vi "AlliGator Get Decay Fit Parameter Map Data.vi"(0 "Multiple Decays Fit Parameters":dbl[][](array[numeric]), 1 "Compute Decay Fit Parameter Map":bool, 2 "Output ROI centers?":bool, 5 "X Resolution":i32, 7 "Y Resolution":i32, 11 "Error In":errorcluster, 12 "Map index":i32, 13 "Selected ROI Array":bool[](array[boolean])) -> (4 "Map Data (V x H)":dbl[][](array[numeric]), 6 "New Map Selected?":bool, 8 "# Filtered ROIs":i32, 10 "ROI Centers":cluster{"X":dbl, "Y":dbl}[](array[cluster]), 15 "Error Out":errorcluster)   [LabVIEW 2021, in "AlliGator Decay Fit Parameter Map.lvlib"]
doc: "Fills in matrix with fit parameter wherever it has been computed, NaN otherwise."
uses:
  AlliGator Decay Fit Parameter Map.lvlib
  Globals, Variables, Constants/AlliGator Variables List.ctl
  Variant/Variant to Data/Variant to Boolean.vi
  <vilib>/Utility/error.llb/Error Cluster From Error Code.vi
  <vilib>/ErrorRing/Error Ring.xnode
  Globals, Variables, Constants/AlliGator Globals, Variables & Constants.lvlib
  Variant/Variant to Data/Variant to Data.lvlib
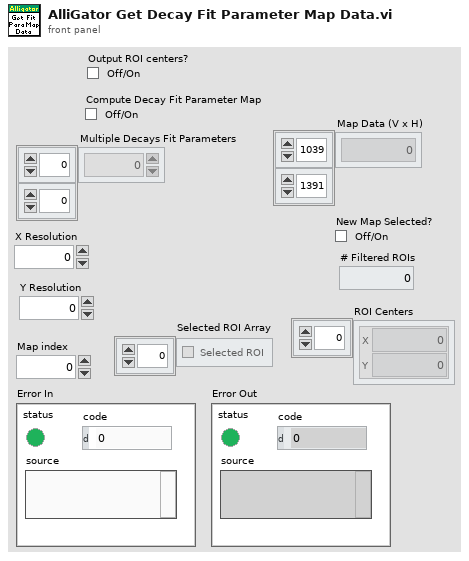
[diagram p1: front panel]
types:
  T1 = typedef "AlliGator Globals, Variables & Constants.lvlib/AlliGator Variables List.ctl" = enum16{"---- GUI ----", "GUI:Initialization Status", "GUI:State Indicators Refnum", "GUI:Original AlliGator Menu Items", "GUI:Current Action Loop State", "GUI:Script in progress", "GUI:Playback", "GUI:Loop Playback", "GUI:Search ROI Used", "GUI:Search ROI", "Decay Graph Max Legend Size", "Intensity Graph Max Legend Size", "Decay Statistics Graph Max Legend Size", "Phasor Graph Max Legend Size", "Phasor Ratio Graph Max Legend Size", "Lifetime Graph Max Legend Size", "---- Files ----", "Files:Export Dataset Frames as Individual Files", "Files:Show Batch Export Help Balloons", "Files:Frames in Dataset", "Files:ptu File Frame Start Indices", "Files:Current Frame in Dataset", "Files:Current Frame Timestamp", "Files:Dataset Loaded", "Files:Dataset Metadata", "Files:Dataset Channel", "Files:Dataset Data Description", "Files:Background Dataset Metadata", "Files:Background Dataset Channel", "Files:Background Dataset Data Description", "Files:Background File Subtraction", "Files:Background File Path", "Files:Background File Pile-up Correction", "Files:Background File Pixel Well Capacity", "Files:Background File Scaling Factor", "Files:Current Dataset Load Settings", "Files:Dataset Path", "Files:ICCD-specific Information", "Files:Macrotime Gate Separation", "------ Python Plugins ------", "Python Plugins:Information", "Python Plugins:Python Session", "Python Plugins:Valid Python Session?", "---- Source Image ----", "Source Image:ROIs", "Source Image:Current ROI", "Source Image:ROI Event Refnum", "X_Source Image:Display Range", "X_Source Image:Palette Information", "X_Source Image:Type of Displayed Image", "X_Time Gate Slider", "Source Image:Palette List", "Source Image:Scale", "Source Image:ROI Overlay Color", "Source Image:Overlay to Erase", "Source Image:Is Displayed Image Accumulated", "Source Image:White Light Image Modified", "Source Image:Mask Image Modified", "---- Image Profile Window ----", "Image Profile:Window Event Refnum", "Image Profile:IntensityType", "Image Profile:Intensity Average Type", "Image Profile:Intensity-weighted SDV", "Image Profile:Box Profile Type", "Image Profile:Window Open", "Image Profile:Plotted Fit Parameter", "------ Phasor Graph -------", "Phasor Graph:Show Line", "---- Phasor Plot ---", "Phasor Plot:Parameters Changed", "Phasor Plot:FLI Dataset Modified since last Calculation", "Phasor Harmonics Data", "Selected Phasor Harmonics", "Phasor Harmonic Manager Event Refnum", "Phasor Plot:ROIs", "Phasor Plot:Current ROI", "Phasor Plot:ROI Event Refnum", "Phasor Plot:Image Reference Points", "Phasor Plot:Computed", "Phasor Plot:Palette Information", "Phasor Plot:Palette List", "Phasor Plot:Phasor Ratio Palette Information", "Phasor Plot:Phasor Ratio Palette List", "Phasor Plot:Image Scale", "Phasor Plot:Image Overlay to Erase", "Phasor Plot:Image Elements to Update", "Phasor Plot:Current Calculation Parameters", "Phasor Plot:Current Calibration Options", "Phasor Plot:Reset Cumulated Phasor Plot", "Phasor Plot:Reference 1", "Phasor Plot:Lifetime Reference 1", "Phasor Plot:Reference 1 Frequency", "Phasor Plot:Reference 2", "Phasor Plot:Lifetime Reference 2", "Phasor Plot:Reference 2 Frequency", "---- Decay Analysis ----", "Number of Selected Decays to Fit", "LS Fit Results", "LAR Fit Results", "BS Fit Results", "Last Decay Max - Min", "Best Fit Parameters", "Best Fit Parameter Names", "Actual Size X", "Actual Size Y", "Binning X", "Binning Y", "Actual # Gates", "Dataset Number", "Gates to...", "Gates Skipped", "Gates to keep", "Gate Step", "Gate Separation", "Reversed Gates", "Pile-up Correction", "Pixel Well Capacity", "Background Subtracted", "Background Subtraction Method", "Background Definition Range", "Background File (deprecated)", "Number of Dataset Accumulated", "Array of Accumulated Dataset Paths", "Do Averaged Datasets", "Destination File Path", "Process Plot Target", "Use 1/D as Phasor Frequency", "---- Decay Fit Parameter Map -----", "Decay Fit Parameter Map:Palette Information", "Decay Fit Parameter Map:Palette List", "Decay Fit Parameter Map:X Resolution", "Decay Fit Parameter Map:Y Resolution", "Decay Fit Parameter Map:Use Decay Fit Result Constraints", "Decay Fit Parameter Map:Decay Fit Result Constraints", "Decay Fit Parameter Map:Decay Fit Result Constraints Applied", "---- Parameter Map ----", "Parameter Map:Palette Information", "Parameter Map:Palette List", "------- Local Decay Window ---------", "Local Decay Graph Window:Event Refnum", "Local Decay Graph Window:Use normalized IRF for convolution", "----- Miscellaneous ----", "Misc:Skippable Dialog Windows Status"}
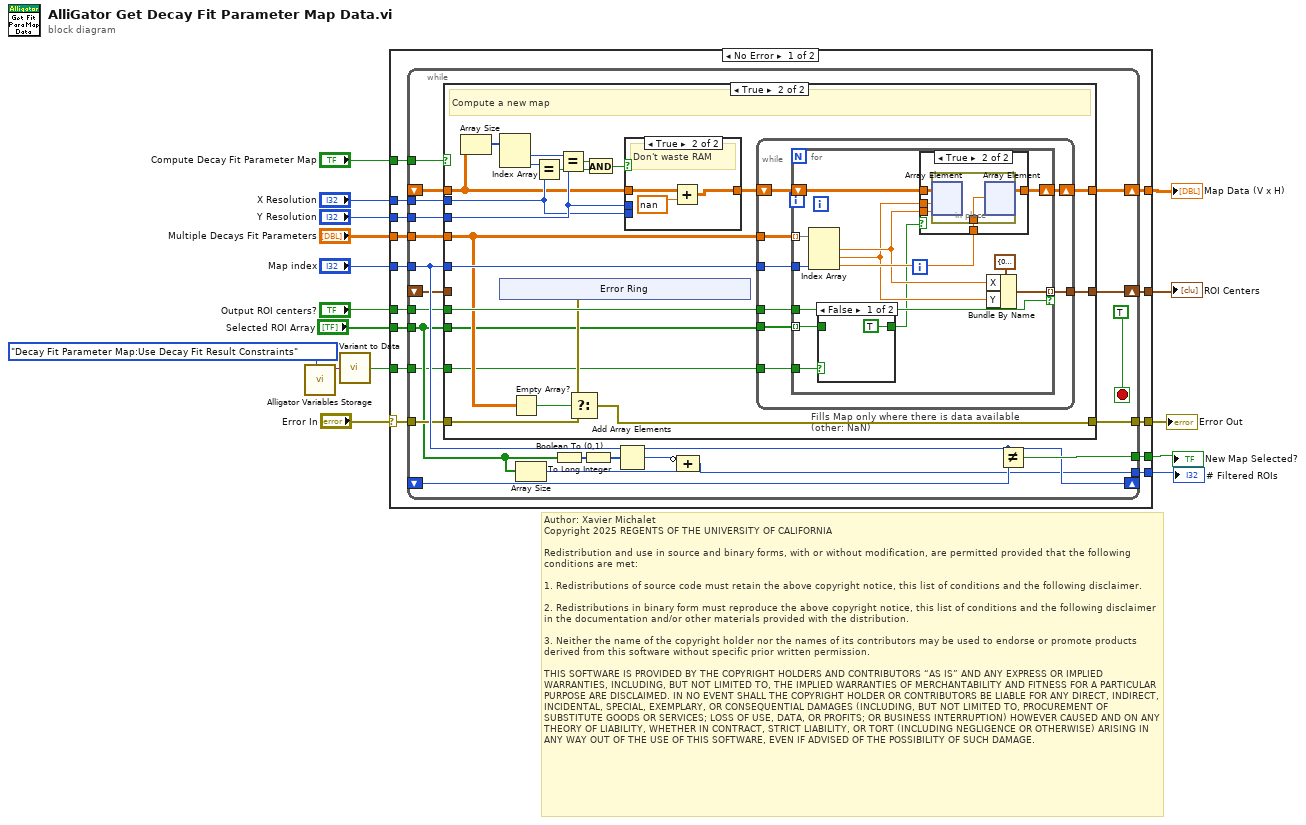
[diagram p0: block diagram]
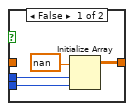
[diagram p5: hidden frame]
diagram:
  # "Author: Xavier Michalet\nCopyright 2025 REGENTS OF THE UNIVERSITY OF CALIFORNIA\n\nRedistribution and use in source and binary forms, with or without modification, are permitted provided that the following conditions are met:\n\n1. Redistributions of source code must retain the above copyright notice, this list of conditions and the following disclaimer.\n\n2. Redistributions in binary form must reproduce the above copyright notice, this list of conditions and the following disclaimer in the documentation and/or other materials provided with the distribution.\n\n3. Neither the name of the copyright holder nor the names of its contributors may be used to endorse or promote products derived from this software without specific prior written permission.\n\nTHIS SOFTWARE IS PROVIDED BY THE COPYRIGHT HOLDERS AND CONTRIBUTORS “AS IS” AND ANY EXPRESS OR IMPLIED WARRANTIES, INCLUDING, BUT NOT LIMITED TO, THE IMPLIED WARRANTIES OF MERCHANTABILITY AND FITNESS FOR A PARTICULAR PURPOSE ARE DISCLAIMED. IN NO EVENT SHALL THE COPYRIGHT HOLDER OR CONTRIBUTORS BE LIABLE FOR ANY DIRECT, INDIRECT, INCIDENTAL, SPECIAL, EXEMPLARY, OR CONSEQUENTIAL DAMAGES (INCLUDING, BUT NOT LIMITED TO, PROCUREMENT OF SUBSTITUTE GOODS OR SERVICES; LOSS OF USE, DATA, OR PROFITS; OR BUSINESS INTERRUPTION) HOWEVER CAUSED AND ON ANY THEORY OF LIABILITY, WHETHER IN CONTRACT, STRICT LIABILITY, OR TORT (INCLUDING NEGLIGENCE OR OTHERWISE) ARISING IN ANY WAY OUT OF THE USE OF THIS SOFTWARE, EVEN IF ADVISED OF THE POSSIBILITY OF SUCH DAMAGE."
  n1 = call "Alligator Variables Storage.vi"("AlliGator Variable"=AlliGator_Variables_List."Decay Fit Parameter Map:Use Decay Fit Result Constraints") -> ("Data out"=w3:variant)  [unwired: 8 in, 2 out]
  n2 = call-poly "Variant to Data.vi"("Variant"=w3) -> ("Value"=w2:bool)  [unwired: 8 in]
  n3 = case shown="No Error" "Error In" {
    selector: "Error In" -> [w21 w119]
    tunnel: "Y Resolution" -> [w30 _]
    tunnel: "X Resolution" -> [w29 _]
    tunnel: "Map index" -> [w28 _]
    tunnel: [w27 _] -> w13
    tunnel: [w26 _] -> w12
    tunnel: "Compute Decay Fit Parameter Map" -> [w25 _]
    tunnel: "Multiple Decays Fit Parameters" -> [w24 _]
    tunnel: [w23 _] -> w8
    tunnel: "Output ROI centers?" -> [w22 _]
    tunnel: [w20 w119] -> w6
    tunnel: "Selected ROI Array" -> [w19 _]
    tunnel: [w18 _] -> w4
    tunnel: w2 -> [w17 _]
    frame No Error {
      n4 = while {
        tunnel: w24 -> [w51]
        tunnel: w25 -> [w50]
        shift-right: [w52] -> w26
        shift-left: _ -> [w48]
        tunnel: w28 -> [w43]
        shift-right: [w43] -> _
        shift-left: _ -> [w47]
        tunnel: [w46] -> w27
        tunnel: w29 -> [w45]
        tunnel: w30 -> [w44]
        tunnel: w22 -> [w41]
        shift-right: [w42] -> w23
        shift-left: _ -> [w40]
        tunnel: w21 -> [w39]
        tunnel: [w38] -> w20
        tunnel: w19 -> [w35]
        tunnel: [w32] -> w18
        tunnel: w17 -> [w31]
        stop <- TRUE stop-if-true
        n5 = case shown="True" w50 {
          tunnel: [w55 w76] -> w52
          tunnel: w51 -> [_ w62]
          tunnel: w48 -> [w55 w63]
          tunnel: w43 -> [_ w74]
          tunnel: w45 -> [_ w67]
          tunnel: w44 -> [_ w69]
          tunnel: [w54 w73] -> w42
          tunnel: w41 -> [_ w72]
          tunnel: w40 -> [w54 _]
          tunnel: w39 -> [w53 w59]
          tunnel: [w53 w58] -> w38
          tunnel: w35 -> [_ w57]
          tunnel: w31 -> [_ w56]
          frame False {
            # "use old map"
          }
          frame True {
            # "Compute a new map"
            n6 = Array Size(array=w63) -> (size(s)=w71:i32[])
            n7 = Index Array(array=w71) -> (element #1=w70:i32, element #2=w68:i32)  [unwired: 2 in]
            n8 = xnode "Error Ring"() -> ("error out"=w60:errorcluster)
            n9 = Empty Array?(array=w62) -> (empty?=w61:bool)
            n10 = Equal?(x=w68, y=w67) -> (x = y?=w65:bool)
            n11 = Equal?(x=w70, y=w69) -> (x = y?=w66:bool)
            n12 = Select(t=w60, s=w61, f=w59) -> (s? t:f=w58:errorcluster)
            n13 = And(x=w66, y=w65) -> (x .and. y?=w64:bool)
            n14 = case shown="True" w64 {
              tunnel: [w114 w116] -> w75
              tunnel: w69 -> [w113 _]
              tunnel: w67 -> [w112 _]
              tunnel: w63 -> [_ w118]
              frame False {
                n15 = Initialize Array(nan, w113, w112) -> (w114:dbl[][])
              }
              frame True {
                # "Don't waste RAM"
                n16 = Add(x=w118, y=nan) -> (x+y=w116:dbl[][])
              }
            }
            n17 = while "Fills Map only where there is data available (other: NaN)" {
              shift-right: [w89] -> w76
              shift-left: w75 -> [w86]
              tunnel: w62 -> [w87]
              tunnel: w74 -> [w85]
              tunnel: [w84] -> w73
              tunnel: w72 -> [w83]
              tunnel: w57 -> [w82]
              tunnel: w56 -> [w81]
              stop <- TRUE stop-if-true
              n18 = for {
                shift-right: [w101] -> w89
                shift-left: w86 -> [w102]
                tunnel: w87 -> [w100] mode=indexing
                tunnel: w85 -> [w99]
                tunnel: [w94] -> w84 mode=indexing if=w93
                tunnel: w83 -> [w93]
                tunnel: w82 -> [w91] mode=indexing
                tunnel: w81 -> [w92]
                n19 = Index Array(array=w100, index #3=w99) -> (element #1=w96:dbl, element #2=w95:dbl, element #3=w98:dbl)  [unwired: 2 in]
                n20 = case shown="False" w92 {
                  tunnel: w91 -> [_ w104]
                  tunnel: [TRUE ("Selected ROI") w104] -> w90
                  frame False {
                  }
                  frame True {
                  }
                }
                n21 = case shown="True" w90 {
                  tunnel: w102 -> [w105 w110]
                  tunnel: [w105 w109] -> w101
                  tunnel: w98 -> [_ w108]
                  tunnel: w96 -> [_ w107]
                  tunnel: w95 -> [_ w106]
                  frame False {
                  }
                  frame True {
                    n22 = in-place {
                      in-place-border: w108 -> [w111]
                      n23 = in-place-array #1(w110, w106, w107) -> ()  [unwired: 1 out]
                      n24 = in-place-array #1(w111) -> (w109:dbl[][])  [unwired: 2 out]
                    }
                  }
                }
                n25 = Bundle By Name(cluster=cluster{"X":dbl, "Y":dbl} {"X"=0.0, "Y"=0.0} ("ROI Centers"), "X"=w96, "Y"=w95) -> (w94:cluster{"X":dbl, "Y":dbl})
              }
            }
          }
        }
        n26 = Array Size(array=w35) -> (size(s)=w33:i32)
        n27 = Boolean To (0,1)(Boolean=w35) -> (0, 1=w37:i16[])
        n28 = To Long Integer(number=w37) -> (32bit integer=w36:i32[])
        n29 = Add Array Elements(numeric array=w36) -> (sum=w34:i32)
        n30 = Compound Arithmetic op=unknown(invert w34, w33) -> (w32:i32)
        n31 = Not Equal?(x=w43, y=w47) -> (x != y?=w46:bool)
      }
    }
    frame Error {
    }
  }
  "New Map Selected?" <- w13
  "Map Data (V x H)" <- w12
  "Error Out" <- w6
  "ROI Centers" <- w8
  "# Filtered ROIs" <- w4
